vi "MarkerEnter.vi"(4 "Ground Station Operations Queue Ref":refnum<queue>, 5 "Event Data":cluster{"item":refnum<k24>}, 6 "Control Ref":refnum<k24>, 7 "Event Common Data":T1) -> ()   [LabVIEW 2014]
uses:
  C:/Robotic Systems/Products/Surveyor/Software/Ground Station/Data/Mapping DLL/GMap.NET.WindowsForms.dll
  Data/Mapping DLL/GMap.NET.WindowsForms.dll
  Application Support/Data Processing Queue/Controls/Data Queue.ctl
  Controls/GMap Marker State.ctl
  FGVs/GMap Marker State/SubVI/Set Marker State.vi
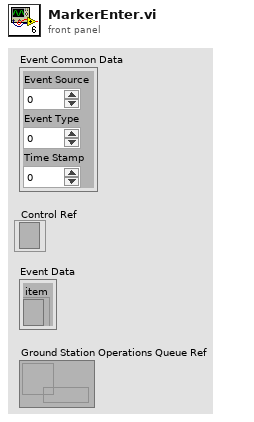
[diagram p1: front panel]
types:
  T1 = cluster{"Event Source":i32, "Event Type":u32, "Time Stamp":u32}
  T2 = typedef "GMap Marker State.ctl" = enum16{"MarkerLeave", "MarkerEntered"}
  T3 = typedef "Data Queue.ctl" = cluster{"Command":string, "Data":variant}
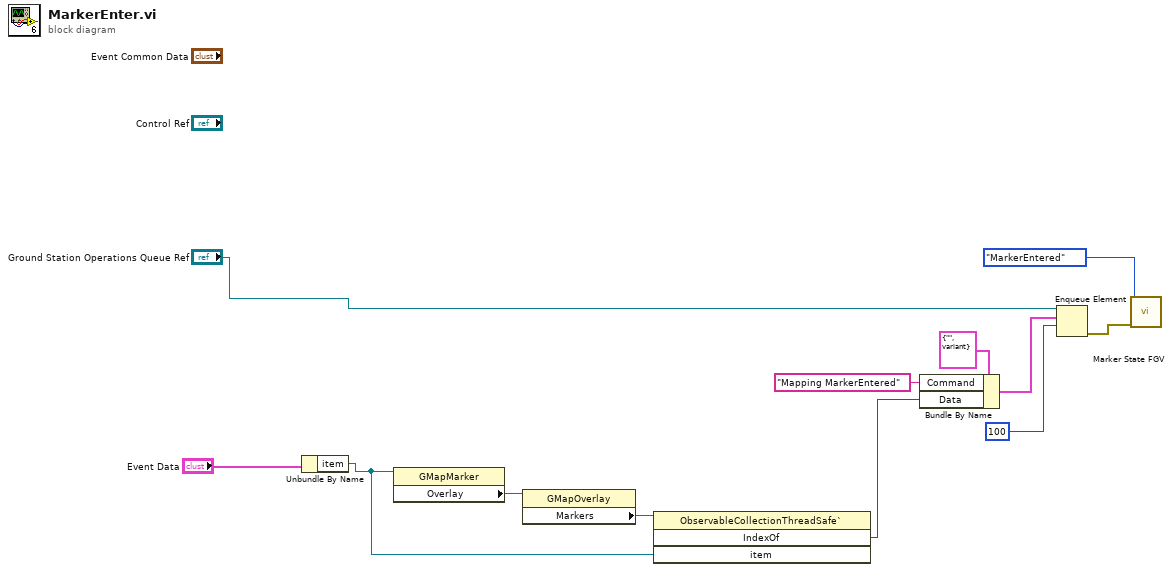
[diagram p0: block diagram]
diagram:
  n1 = Unbundle By Name("Event Data") -> ("item"=w8:refnum<k24>)
  n2 = property class="GMapMarker"(reference=w8) -> ("Overlay"=w10:refnum<k24>)  [unwired: 1 in, 2 out]
  n3 = property class="GMapOverlay"(reference=w10) -> ("Markers"=w9:refnum<k24>)  [unwired: 1 in, 2 out]
  n4 = invoke class="ObservableCollectionThreadSafe`" method="IndexOf"(reference=w9, "item"=w8) -> ("IndexOf"=w7:i32)  [unwired: 2 in, 3 out]
  n5 = Bundle By Name(cluster=T3 {"Command"="", "Data"=variant} ("element"), "Command"="Mapping MarkerEntered", "Data"=w7) -> (w11:T3)
  n6 = Enqueue Element(queue="Ground Station Operations Queue Ref", element=w11, timeout in ms (-1)=100) -> (error out=w2:errorcluster)  [unwired: 1 in, 2 out]
  n7 = call-poly "Marker State FGV.vi"("Error In"=w2, "Marker State In"=GMap_Marker_State."MarkerEntered") -> ()  [unwired: 9 in, 1 out]
